vi "RT Loop - Log Camera Data.vi"(8 "error in (no error)":errorcluster, 10 "RT Video fifo":refnum<k33>, 11 "Queue in":refnum<queue>) -> (3 "Acceleration Log Folder":path=path "/home/lvuser/Log/logfiles_deploy")   [LabVIEW 2017]
uses:
  <vilib>/vision/Image Controls.llb/IMAQ Image.ctl
  UI Error Handlers/support/Message Queue/Message Cluster.ctl
  Globals/Global - All RT Loop Stop.vi
  Globals/Global - Configuration Options.vi
  UI Error Handlers/support/Message Queue/Message Queue.lvlib
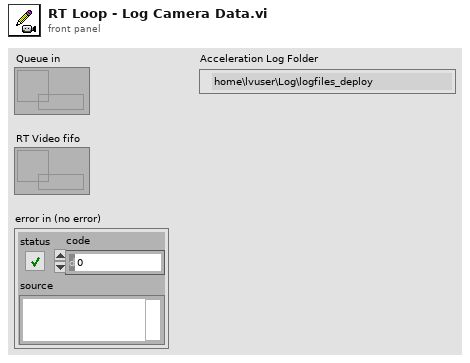
[diagram p1: front panel]
types:
  T1 = typedef "IMAQ Image.ctl" = refnum<image>
  T2 = typedef "IMAQ AVI2 Refnum.ctl" = refnum<k20>
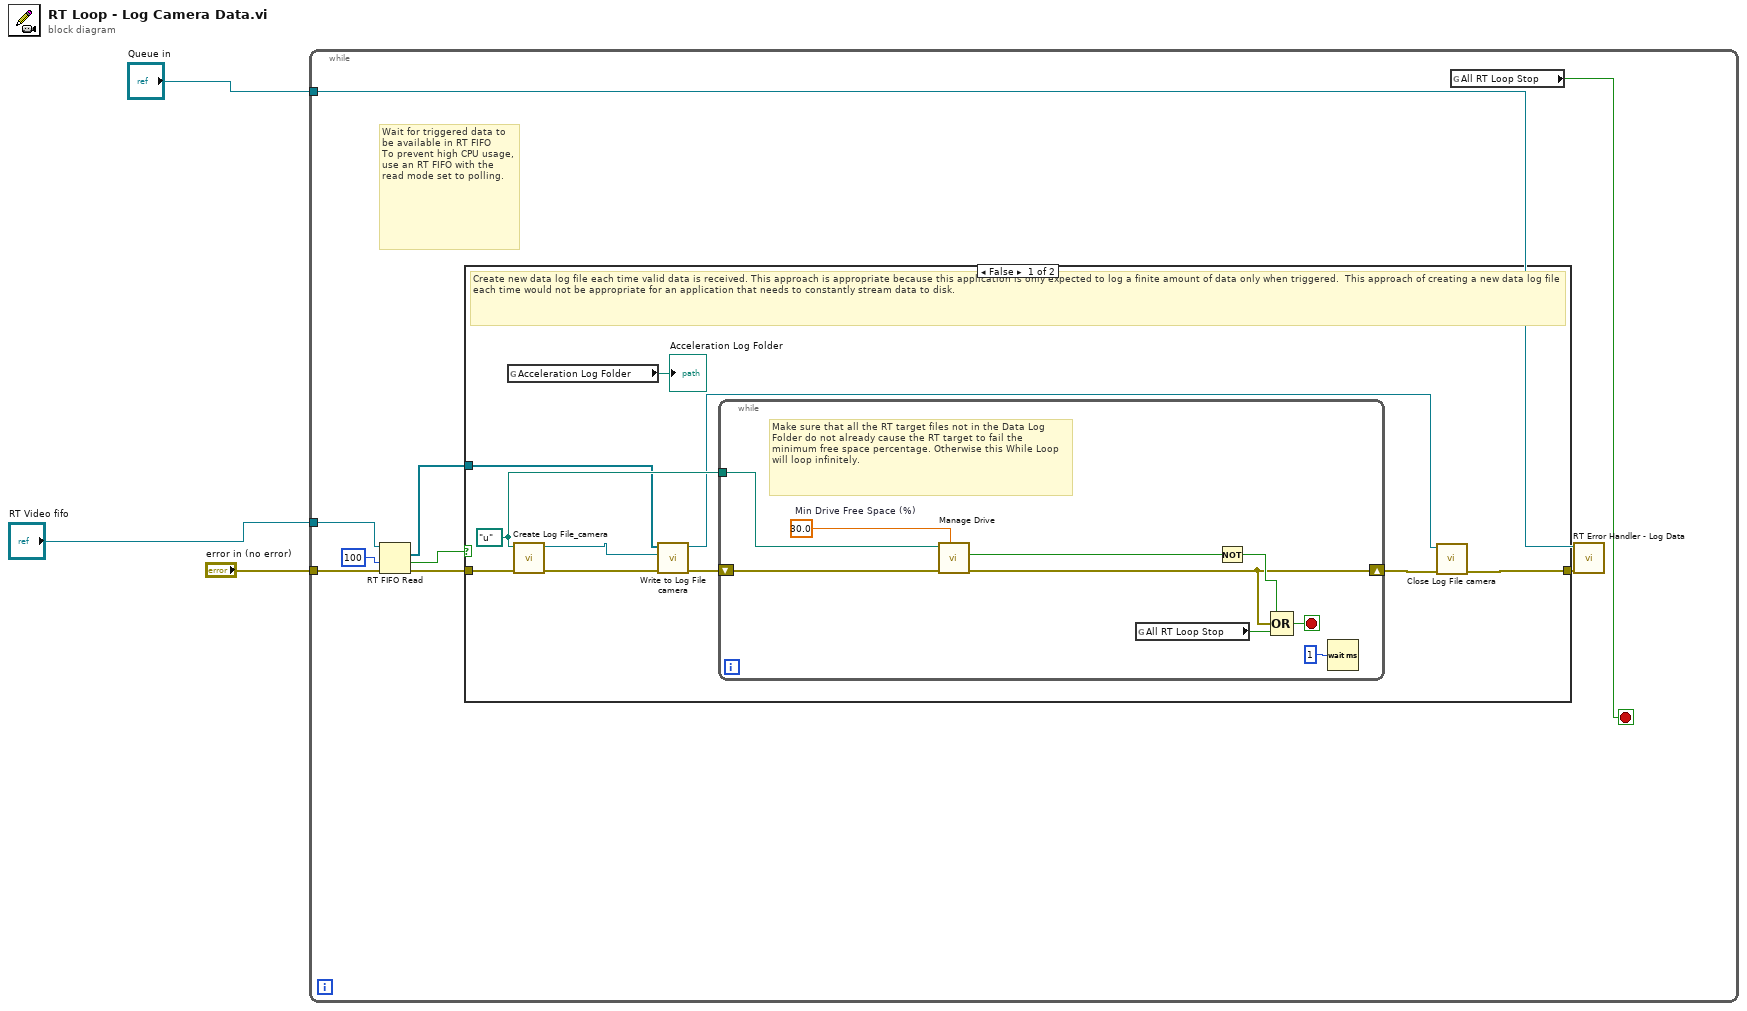
[diagram p0: block diagram]
diagram:
  n1 = while {
    tunnel: "RT Video fifo" -> [w10]
    tunnel: "Queue in" -> [w7]
    tunnel: "error in (no error)" -> [w12]
    stop <- w8 stop-if-true
    # "Wait for triggered data to be available in RT FIFO\nTo prevent high CPU usage, use an RT FIFO with the read mode set to polling."
    n2 = RT FIFO Read(0:w10, 2:100 ("ms timeout (0)"), 3:w12) -> (9:w9:T1[], 10:w4:bool, 11:w11:errorcluster)  [unwired: 1 in, 2 out]
    n3 = case shown="False" w4 {
      tunnel: w9 -> [w14 _]
      tunnel: w11 -> [w18 w32]
      tunnel: [w20 w32] -> w6
      frame False {
        w17 = path "u:/" ("file path (use dialog)")
        # "Create new data log file each time valid data is received. This approach is appropriate because this application is only expected to log a finite amount of data only when triggered.  This approach of creating a new data log file each time would not be appropriate for an application that needs to constantly stream data to disk."
        n4 = global read "Global - Configuration Options.vi" "Acceleration Log Folder"() -> (→"Acceleration Log Folder":path)
        n5 = call "Create Log File_camera.vi"("error in (no error)"=w18, "Acceleration Exceeded Log Folder"=w17) -> ("error out"=w19:errorcluster, "AVI Refnum"=w13:T2)  [unwired: 8 in]
        n6 = call "Write to Log File camera.vi"("error in (no error)"=w19, "AVI Refnum in"=w13, "Array"=w14) -> ("error out"=w22:errorcluster, "AVI Refnum output"=w15:T2)  [unwired: 7 in]
        n7 = while {
          shift-right: [w26] -> w21
          shift-left: w22 -> [w27]
          tunnel: w17 -> [w24]
          stop <- w31 stop-if-true
          w25 = 30.0  # Min Drive Free Space (%)
          # "Make sure that all the RT target files not in the Data Log Folder do not already cause the RT target to fail the minimum free space percentage. Otherwise this While Loop will loop infinitely."
          n8 = call "Manage Drive.vi"("Min Drive Free Space (%)"=w25, "error in"=w27, "Data Folder"=w24) -> ("error out"=w26:errorcluster, "Drive Space Below Limit"=w23:bool)  [unwired: 7 in]
          n9 = global read "Global - All RT Loop Stop.vi" "All RT Loop Stop"() -> (w28:bool)
          n10 = Not(x=w23) -> (.not. x?=w30:bool)
          n11 = Compound Arithmetic op=OR(w30, w26, w28) -> (w31:bool)
          n12 = Wait (ms)(milliseconds to wait=u32 1) -> ()  [unwired: 1 out]
        }
        n13 = call "Close Log File camera.vi"("error in (no error)"=w21, "AVI Refnum in"=w15) -> ("error out"=w20:errorcluster)  [unwired: 9 in]
      }
      frame True {
        # "Timed out - No data"
      }
    }
    n14 = global read "Global - All RT Loop Stop.vi" "All RT Loop Stop"() -> (w8:bool)
    n15 = call "RT Error Handler - Log Data.vi"("error in (no error)"=w6, "Message Queue"=w7) -> ()  [unwired: 9 in, 1 out]
  }
